vi "ResetFactoryDefaults.vi"(8 "error in (no error)":errorcluster, 10 "Address":u8, 11 "VISA resource name":refnum<visa-resource-name>) -> (0 "error out":errorcluster, 1 "Raw Response":string, 3 "VISA resource name out":refnum<visa-resource-name>)   [LabVIEW 2020, in "driver_flodx_pressure.lvlib"]
doc: "Must be in CONFIG mode."
uses:
  <instrlib>/RxnRover/FloDx Pressure Driver/driver_flodx_pressure.lvlib
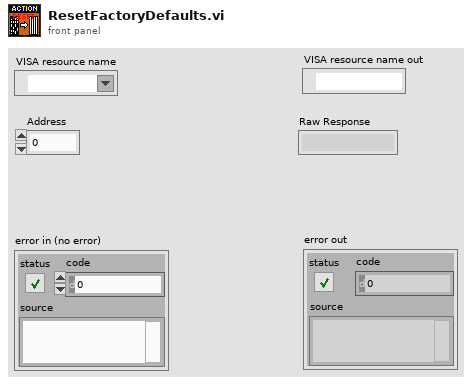
[diagram p1: front panel]
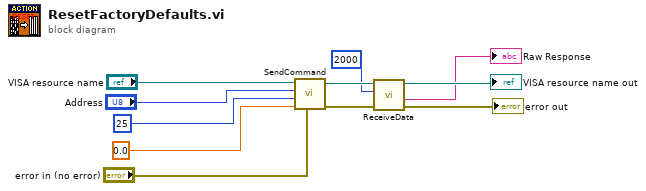
[diagram p0: block diagram]
diagram:
  n1 = call <instrlib>:"SendCommand.vi"("error in"="error in (no error)", "Parameter"=sgl 0.0 ("Address(New)"), "Command"=u8 25, "Address"="Address", "VISA resource name"="VISA resource name") -> ("error out"=w6:errorcluster, "VISA resource name out"=w2:refnum<visa-resource-name>)  [unwired: 4 in, 1 out]
  n2 = call <instrlib>:"ReceiveData.vi"("error in (no error)"=w6, "Delay before read (ms)"=u32 2000, "VISA resource name"=w2) -> ("error out"=→"error out":errorcluster, "Raw Response"=→"Raw Response":string, "VISA resource name out"=→"VISA resource name out":refnum<visa-resource-name>)  [unwired: 4 in, 2 out]
